vi "SubVI Tester.vi"() -> ()   [LabVIEW 2017]
uses:
  Weather Data.ctl
panel:
  out "Weather Data Out":T1={"Current Temperature"=0.0, "Max Temperature"=0.0, "Min Temperature"=0.0, "Temperature Warning Text"="No Warning", "Temperature Warning?"=FALSE, "Current Windspeed"=0.0, "Max Windspeed"=0.0, "Windspeed Warning?"=FALSE, "Windspeed Warning Text"=""}
  in  "Weather Data In":T1={"Current Temperature"=0.0, "Max Temperature"=0.0, "Min Temperature"=0.0, "Temperature Warning Text"="No Warning", "Temperature Warning?"=FALSE, "Current Windspeed"=0.0, "Max Windspeed"=0.0, "Windspeed Warning?"=FALSE, "Windspeed Warning Text"=""}
  in  "Min Temperature":dbl=10.0
  in  "Max Temperature":dbl=30.0
  in  "Stop":bool
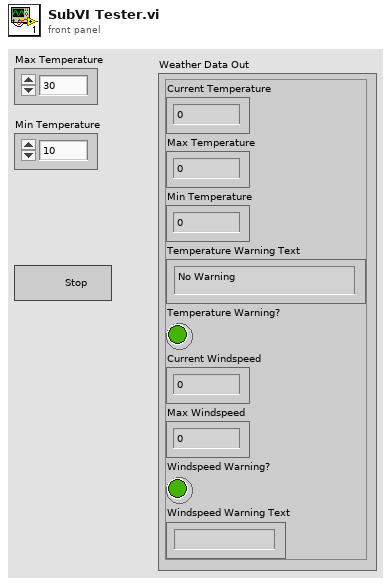
[diagram p1: front panel]
types:
  T1 = typedef "Weather Data.ctl" = cluster{"Current Temperature":dbl, "Max Temperature":dbl, "Min Temperature":dbl, "Temperature Warning Text":string, "Temperature Warning?":bool, "Current Windspeed":dbl, "Max Windspeed":dbl, "Windspeed Warning?":bool, "Windspeed Warning Text":string}
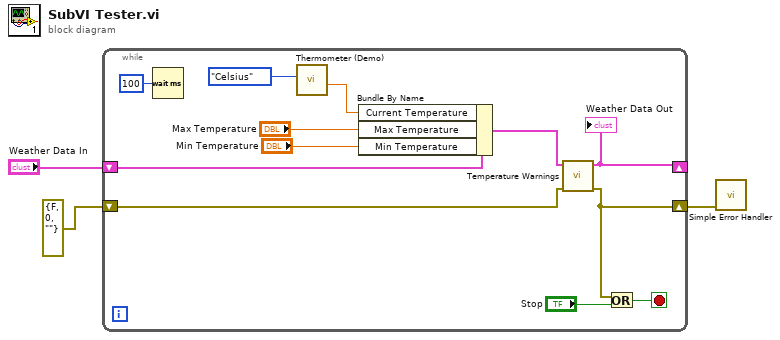
[diagram p0: block diagram]
diagram:
  n1 = while {
    shift-right: [w5] -> w3
    shift-left: errorcluster {"status"=FALSE, "code"=0, "source"=""} ("error in") -> [w6]
    shift-right: [w4] -> _
    shift-left: "Weather Data In" -> [w11]
    stop <- w13 stop-if-true
    n2 = Wait (ms)(milliseconds to wait=u32 100) -> ()  [unwired: 1 out]
    n3 = call "Thermometer (Demo).vi"("Units (0: Celsius)"=enum16{"Celsius"}."Celsius") -> ("Temperature Value"=w10:dbl)  [unwired: 10 in]
    n4 = Bundle By Name(cluster=w11, "Current Temperature"=w10, "Max Temperature"="Max Temperature", "Min Temperature"="Min Temperature") -> (w7:T1)
    n5 = call "Temperature Warnings.vi"("Error In"=w6, "Weather Data In"=w7) -> ("Error Out"=w5:errorcluster, "Weather Data Out"=w4:T1)  [unwired: 8 in]
    "Weather Data Out" <- w4
    n6 = Or(x=w5, y="Stop") -> (x .or. y?=w13:bool)
  }
  n7 = call <vilib>:"Simple Error Handler.vi"("error in (no error)"=w3) -> ()  [unwired: 4 in, 5 out]
